vi "FloatArrayToStringArray.vi"(1 "测试结果":dbl[](array[numeric])) -> (0 "String数组":string[](array[string]))   [LabVIEW 2014]
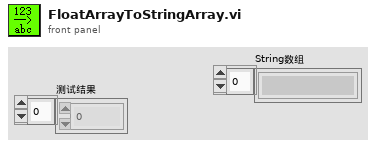
[diagram p1: front panel]
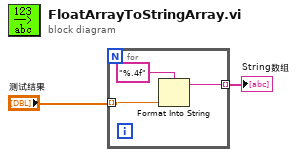
[diagram p0: block diagram]
diagram:
  n1 = for {
    tunnel: "测试结果" -> [w5] mode=indexing
    tunnel: [w4] -> w1 mode=indexing
    n2 = Format Into String(format string="%.4f" ("初始字符串"), w5) -> (resulting string=w4:string)  [unwired: 2 in, 1 out]
  }
  "String数组" <- w1
